vi "Update Parameters Values.vi"(8 "error in":errorcluster, 9 "record in":T1 {"type" format="%04x"; "activity" format="%04x"; "error" format="%04x"; "cwd1" format="%04x"; "cwd2" format="%04x"; "swd1" format="%04x"; "swd2" format="%04x"; "data" format="%04x"}, 10 "values in":dbl[](array[numeric]), 11 "Rx execution unit in":refnum<class "Rx Execution Unit.lvclass">) -> (0 "error out":errorcluster, 1 "status error counts":T2, 2 "values out":dbl[](array[numeric]), 3 "Rx execution unit out":refnum<class "Rx Execution Unit.lvclass">)   [LabVIEW 2020, in "Ballard MIL-STD-1553 Engine.lvlib" / "Implementation.lvlib" / "Rx Execution Unit.lvclass"]
uses:
  Rx Execution Unit.lvclass
  Status Error Counts.ctl
  <instrlib>/BTICardLib/Public/Controls/1553 Record.ctl
  <instrlib>/BTICardLib/BTICardLV.lvlib
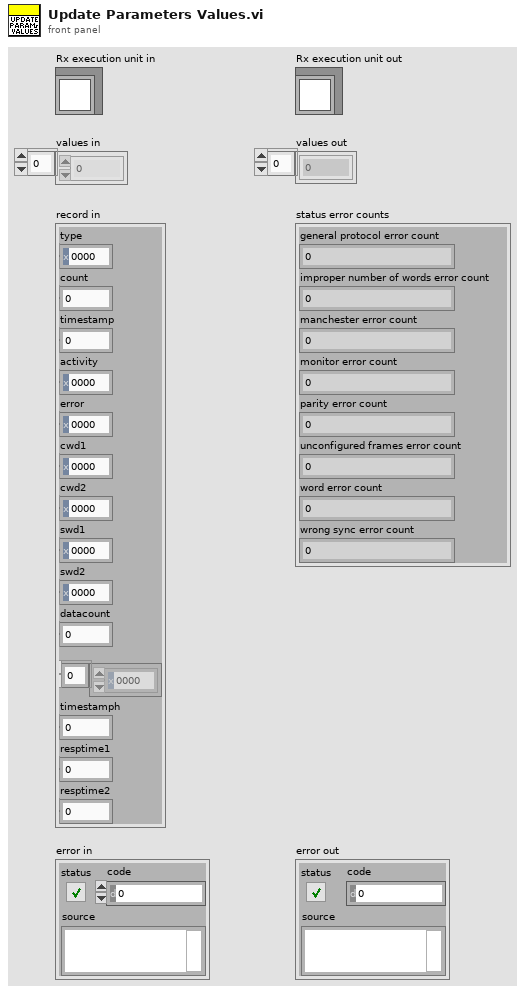
[diagram p1: front panel]
types:
  T1 = typedef "BTICardLV.lvlib/1553 Record.ctl" = cluster{"type":u16, "count":u16, "timestamp":u32, "activity":u16, "error":u16, "cwd1":u16, "cwd2":u16, "swd1":u16, "swd2":u16, "datacount":u16, "data":u16[], "timestamph":u32, "resptime1":u16, "resptime2":u16}
  T2 = typedef "Ballard MIL-STD-1553 Engine.lvlib/Implementation.lvlib/Rx Execution Unit.lvclass/Status Error Counts.ctl" = cluster{"general protocol error count":u64, "improper number of words error count":u64, "manchester error count":u64, "monitor error count":u64, "parity error count":u64, "unconfigured frames error count":u64, "word error count":u64, "wrong sync error count":u64}
  T3 = typedef "Ballard MIL-STD-1553 Engine.lvlib/Implementation.lvlib/Rx Execution Unit.lvclass/Status Terminal Lookup Data.ctl" = cluster{"value index":i32, "remote terminal handle":u64, "terminal address":u64}
  T4 = typedef "Map of Messages to Value Indexes.ctl" = map{T5, T6}
  T5 = typedef "Message Map Key.ctl" = cluster{"HW channel":u16, "terminal address":u16, "subaddress":u16, "mode code":u16}
  T6 = typedef "Ballard MIL-STD-1553 Engine.lvlib/Implementation.lvlib/Rx Execution Unit.lvclass/Message Map Value.ctl" = cluster{"value indexes":i32[], "message":T7, "Tx status count":i32, "Rx status count":i32}
  T7 = typedef "Message Definition.ctl" = cluster{"name":string, "message type":T8, "endpoint Tx":T9, "endpoint Rx":T9, "create timestamp channel":bool, "mode code":u16, "number of words":u16, "parameters":cluster{"name":string, "default value":dbl, "unit":string, "parameter definition":T11}[]}
  T8 = typedef "Message Type.ctl" = string
  T9 = typedef "Terminal Endpoint.ctl" = cluster{"terminal address":T10, "subaddress":T10}
  T10 = typedef "Address.ctl" = u16
  T11 = typedef "Parameter Definition.ctl" = cluster{"start index":i32, "size (bits)":i32, "encoding":enum16{"BNR", "BCD", "Discrete"}, "signed":bool, "multiplier":dbl, "offset":dbl}
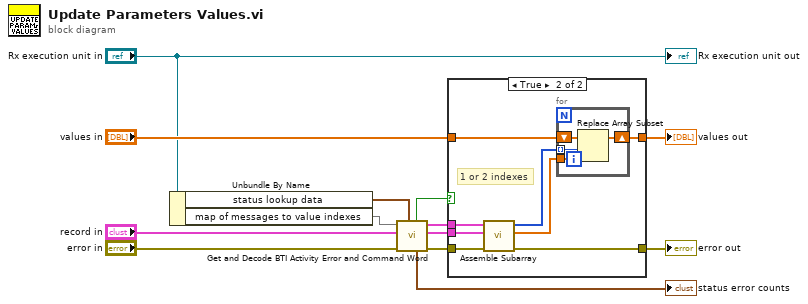
[diagram p0: block diagram]
diagram:
  n1 = Unbundle By Name("Rx execution unit in") -> ("status lookup data"=w1:T3[], "map of messages to value indexes"=w13:T4)
  n2 = call "Get and Decode BTI Activity Error and Command Word.vi"("status lookup data"=w1, "error in"="error in", "record in"="record in", "map of messages to value indexes"=w13) -> ("error out"=w6:errorcluster, "record out"=w10:T1, "value"=w9:T6, "status error counts"=→"status error counts":T2, "update values"=w11:bool)  [unwired: 3 in]
  n3 = case shown="True" w11 {
    tunnel: "values in" -> [w15 w23]
    tunnel: w6 -> [w14 w17]
    tunnel: [w14 w22] -> w4
    tunnel: [w15 w21] -> w7
    tunnel: w9 -> [_ w18]
    tunnel: w10 -> [_ w16]
    frame False {
    }
    frame True {
      # "1 or 2 indexes"
      n4 = call "Assemble Subarray.vi"("error in"=w17, "Rx record"=w16, "message"=w18) -> ("error out"=w22:errorcluster, "subarray"=w19:dbl[], "value indexes"=w20:i32[])  [unwired: 6 in]
      n5 = for {
        shift-right: [w27] -> w21
        shift-left: w23 -> [w26]
        tunnel: w20 -> [w25] mode=indexing
        tunnel: w19 -> [w24]
        # "For Each value index"
        n6 = Replace Array Subset(array=w26, new element=w24, index=w25) -> (w27:dbl[])
      }
    }
  }
  "values out" <- w7
  "error out" <- w4
  "Rx execution unit out" <- "Rx execution unit in"
